vi "Start Sync.vi"(8 "error in (no error)":errorcluster, 11 "gRPC Server in":refnum<class "GreeterService.lvclass">) -> (0 "error out":errorcluster, 3 "gRPC Server out":refnum<class "GreeterService.lvclass">)   [LabVIEW 2019, in "Generated_server.lvlib" / "GreeterService.lvclass"]
uses:
  GreeterService.lvclass
  GreeterService.lvclass/GreeterService.ctl
  RPC Messages/Greeter_res.ctl
  RPC Messages/Greeter_res_res_oneof/Greeter_res_res_oneof.lvclass
  RPC Messages/Greeter_req_req_oneof/Greeter_req_req_oneof.lvclass/Greeter_req_req_oneof.ctl
  RPC Messages/Greeter_res_res_oneof/Greeter_res_res_oneof.lvclass/Greeter_res_res_oneof.ctl
  Generated_server.lvlib
  RPC Messages/Greeter_req_req_oneof/Greeter_req_req_oneof.lvclass
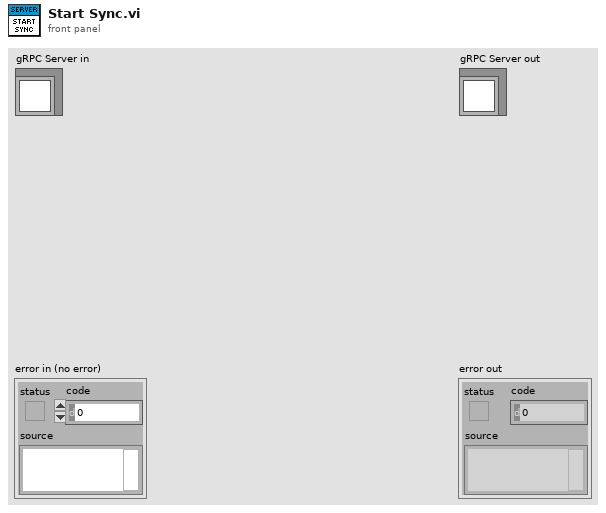
[diagram p1: front panel]
types:
  T1 = typedef "Generated_server.lvlib/Greeter_res.ctl" = cluster{"res_latitude":i32, "Greeter_res_res_oneof":refnum<class "Greeter_res_res_oneof.lvclass">}
  T2 = typedef "Generated_server.lvlib/GreeterService.lvclass/Server Internal UEs.ctl" = cluster{"GreeterService GetFeature Internal UE":refnum<user-event>}
  T3 = typedef "Generated_server.lvlib/GreeterService.lvclass/Server gRPC UEs.ctl" = cluster{"GreeterService GetFeature gRPC UE":refnum<user-event>}
  T4 = typedef "grpc-lvsupport-release.lvlib/grpcId.ctl" = u64
  T5 = typedef "Generated_server.lvlib/Greeter_req.ctl" = cluster{"req_latitude":i32, "Greeter_req_req_oneof":refnum<class "Greeter_req_req_oneof.lvclass">}
  T6 = typedef "grpc-lvsupport.lvlib/grpcId.ctl" = u64
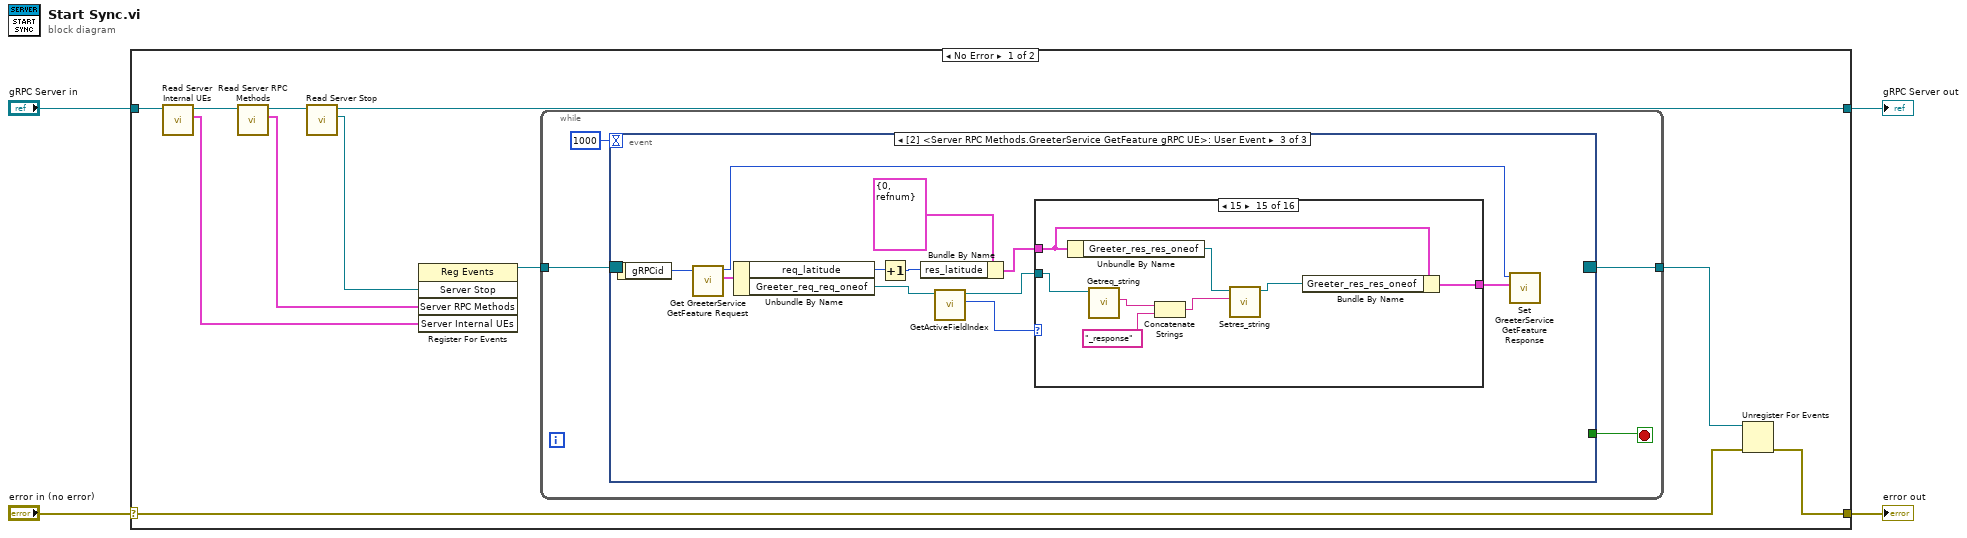
[diagram p0: block diagram]
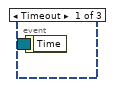
[diagram p2: hidden frame]
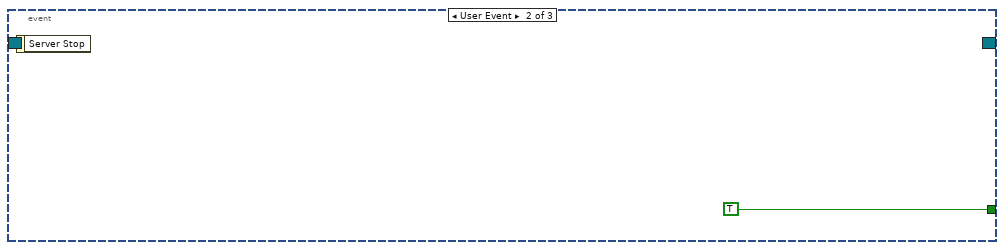
[diagram p3: hidden frame]
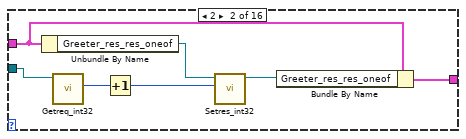
[diagram p5: hidden frame]
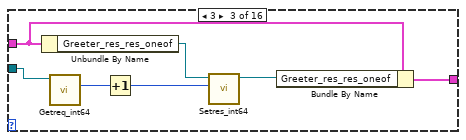
[diagram p6: hidden frame]
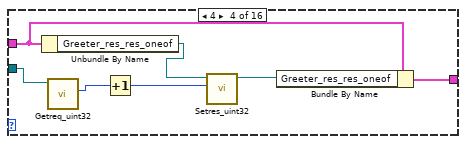
[diagram p7: hidden frame]
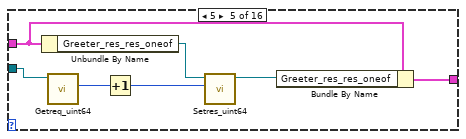
[diagram p8: hidden frame]
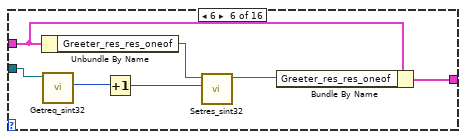
[diagram p9: hidden frame]
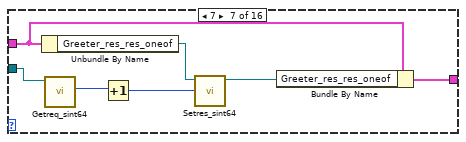
[diagram p10: hidden frame]
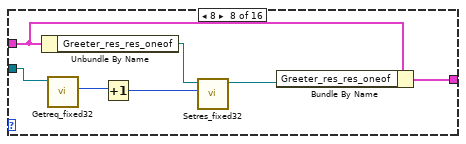
[diagram p11: hidden frame]
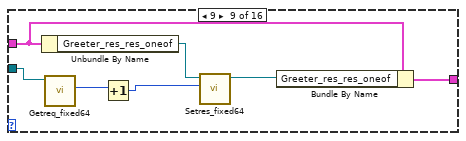
[diagram p12: hidden frame]
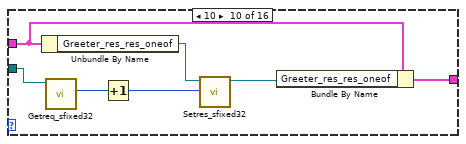
[diagram p13: hidden frame]
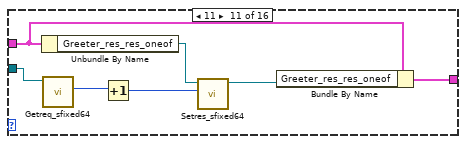
[diagram p14: hidden frame]
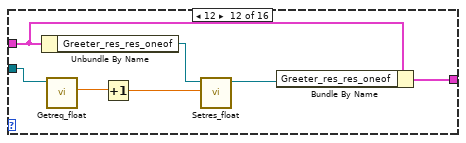
[diagram p15: hidden frame]
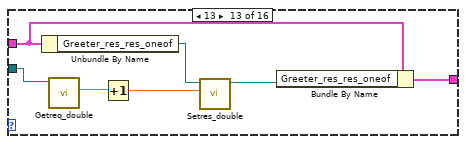
[diagram p16: hidden frame]
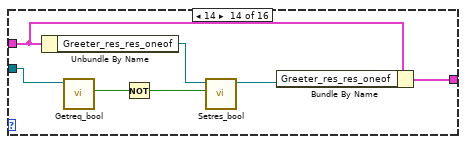
[diagram p17: hidden frame]
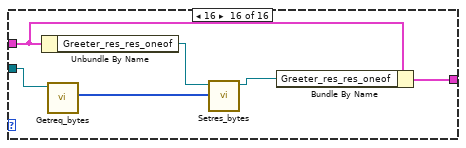
[diagram p18: hidden frame]
diagram:
  n1 = case shown="No Error" "error in (no error)" {
    selector: "error in (no error)" -> [w9 w139]
    tunnel: [w8 w139] -> w3
    tunnel: [w6 w138] -> w1
    tunnel: "gRPC Server in" -> [w15 w138]
    frame No Error {
      n2 = call "Read Server Internal UEs.vi"("SignalGeneratorService in"=w15) -> ("Server Internal UEs"=w13:T2, "SignalGeneratorService out"=w14:refnum<class "GreeterService.lvclass">)  [unwired: 8 in, 1 out]
      n3 = call "Read Server RPC Methods.vi"("SignalGeneratorService in"=w14) -> ("Server RPC Methods"=w7:T3, "SignalGeneratorService out"=w12:refnum<class "GreeterService.lvclass">)  [unwired: 8 in, 1 out]
      n4 = call-dynamic "Read Server Stop.vi"("iService in"=w12) -> ("Server Stop"=w5:refnum<user-event>, "iService out"=w6:refnum<class "GreeterService.lvclass">)  [unwired: 8 in, 1 out]
      n5 = register-events(w5, w7, w13) -> (reference out=w11:refnum<event-registration>)  [unwired: 2 in, 1 out]
      n6 = while {
        tunnel: w11 -> [w19]
        tunnel: [w17] -> w10
        stop <- w18 stop-if-true
        n7 = event "RPC Methods Event Structure" shown="[2] <Server RPC Methods.GreeterService GetFeature gRPC UE>: User Event" {
          selector: w19 -> [_ _ _]
          dyn-events: [_ _ _] -> w17
          timeout: 1000 -> [_ _ _]
          tunnel: [_ TRUE _] -> w18
          event Timeout {
            n8 = event-data() -> ()  [unwired: 1 in, 1 out]
          }
          event User Event {
            n9 = event-data() -> ()  [unwired: 1 in, 1 out]
          }
          event User Event {
            n10 = event-data() -> ("gRPCid"=w31:T4)  [unwired: 1 in]
            n11 = call "Get GreeterService GetFeature Request.vi"("gRPCid in"=w31) -> ("Message Data"=w30:T5, "gRPCid out"=w21:T6)  [unwired: 8 in, 1 out]
            n12 = Unbundle By Name(w30) -> ("req_latitude"=w27:i32, "Greeter_req_req_oneof"=w26:refnum<class "Greeter_req_req_oneof.lvclass">)
            n13 = Increment(x=w27) -> (x+1=w28:i32)
            n14 = Bundle By Name(cluster=T1 {"res_latitude"=0, "Greeter_res_res_oneof"=refnum} ("Greeter_res"), "res_latitude"=w28) -> (w24:T1)
            n15 = call "GetActiveFieldIndex.vi"("OneOfTemplate in"=w26) -> ("Active Field Index"=w25:i32, "OneOfTemplate out"=w23:refnum<class "Greeter_req_req_oneof.lvclass">)  [unwired: 8 in, 1 out]
            n16 = case shown="15" w25 {
              tunnel: w24 -> [w32 w35 w46 w53 w60 w67 w74 w81 w88 w95 w102 w109 w116 w123 w131 w137]
              tunnel: w23 -> [_ w39 w44 w51 w58 w65 w72 w79 w86 w93 w98 w107 w114 w121 w129 w135]
              tunnel: [w32 w33 w45 w52 w59 w66 w73 w80 w87 w94 w101 w108 w115 w122 w130 w136] -> w22
              frame 0, Default {
              }
              frame 2 {
                n17 = Unbundle By Name(w35) -> ("Greeter_res_res_oneof"=w36:refnum<class "Greeter_res_res_oneof.lvclass">)
                n18 = call "Getreq_int32.vi"("OneOfTemplate in"=w39) -> ("Get_Val"=w38:i32)  [unwired: 8 in, 2 out]
                n19 = Increment(x=w38) -> (x+1=w37:i32)
                n20 = call "Setres_int32.vi"("Set_Val"=w37, "OneOfTemplate in"=w36) -> ("OneOfTemplate out"=w34:refnum<class "Greeter_res_res_oneof.lvclass">)  [unwired: 8 in, 1 out]
                n21 = Bundle By Name(cluster=w35, "Greeter_res_res_oneof"=w34) -> (w33:T1)
              }
              frame 3 {
                n22 = Unbundle By Name(w46) -> ("Greeter_res_res_oneof"=w42:refnum<class "Greeter_res_res_oneof.lvclass">)
                n23 = call "Getreq_int64.vi"("OneOfTemplate in"=w44) -> ("Get_Val"=w43:i64)  [unwired: 8 in, 2 out]
                n24 = Increment(x=w43) -> (x+1=w41:i64)
                n25 = call "Setres_int64.vi"("Set_Val"=w41, "OneOfTemplate in"=w42) -> ("OneOfTemplate out"=w40:refnum<class "Greeter_res_res_oneof.lvclass">)  [unwired: 8 in, 1 out]
                n26 = Bundle By Name(cluster=w46, "Greeter_res_res_oneof"=w40) -> (w45:T1)
              }
              frame 4 {
                n27 = Unbundle By Name(w53) -> ("Greeter_res_res_oneof"=w48:refnum<class "Greeter_res_res_oneof.lvclass">)
                n28 = call "Getreq_uint32.vi"("OneOfTemplate in"=w51) -> ("Get_Val"=w50:u32)  [unwired: 8 in, 2 out]
                n29 = Increment(x=w50) -> (x+1=w49:u32)
                n30 = call "Setres_uint32.vi"("Set_Val"=w49, "OneOfTemplate in"=w48) -> ("OneOfTemplate out"=w47:refnum<class "Greeter_res_res_oneof.lvclass">)  [unwired: 8 in, 1 out]
                n31 = Bundle By Name(cluster=w53, "Greeter_res_res_oneof"=w47) -> (w52:T1)
              }
              frame 5 {
                n32 = Unbundle By Name(w60) -> ("Greeter_res_res_oneof"=w55:refnum<class "Greeter_res_res_oneof.lvclass">)
                n33 = call "Getreq_uint64.vi"("OneOfTemplate in"=w58) -> ("Get_Val"=w57:u64)  [unwired: 8 in, 2 out]
                n34 = Increment(x=w57) -> (x+1=w56:u64)
                n35 = call "Setres_uint64.vi"("Set_Val"=w56, "OneOfTemplate in"=w55) -> ("OneOfTemplate out"=w54:refnum<class "Greeter_res_res_oneof.lvclass">)  [unwired: 8 in, 1 out]
                n36 = Bundle By Name(cluster=w60, "Greeter_res_res_oneof"=w54) -> (w59:T1)
              }
              frame 6 {
                n37 = Unbundle By Name(w67) -> ("Greeter_res_res_oneof"=w62:refnum<class "Greeter_res_res_oneof.lvclass">)
                n38 = call "Getreq_sint32.vi"("OneOfTemplate in"=w65) -> ("Get_Val"=w64:i32)  [unwired: 8 in, 2 out]
                n39 = Increment(x=w64) -> (x+1=w63:i32)
                n40 = call "Setres_sint32.vi"("Set_Val"=w63, "OneOfTemplate in"=w62) -> ("OneOfTemplate out"=w61:refnum<class "Greeter_res_res_oneof.lvclass">)  [unwired: 8 in, 1 out]
                n41 = Bundle By Name(cluster=w67, "Greeter_res_res_oneof"=w61) -> (w66:T1)
              }
              frame 7 {
                n42 = Unbundle By Name(w74) -> ("Greeter_res_res_oneof"=w69:refnum<class "Greeter_res_res_oneof.lvclass">)
                n43 = call "Getreq_sint64.vi"("OneOfTemplate in"=w72) -> ("Get_Val"=w71:i64)  [unwired: 8 in, 2 out]
                n44 = Increment(x=w71) -> (x+1=w70:i64)
                n45 = call "Setres_sint64.vi"("Set_Val"=w70, "OneOfTemplate in"=w69) -> ("OneOfTemplate out"=w68:refnum<class "Greeter_res_res_oneof.lvclass">)  [unwired: 8 in, 1 out]
                n46 = Bundle By Name(cluster=w74, "Greeter_res_res_oneof"=w68) -> (w73:T1)
              }
              frame 8 {
                n47 = Unbundle By Name(w81) -> ("Greeter_res_res_oneof"=w76:refnum<class "Greeter_res_res_oneof.lvclass">)
                n48 = call "Getreq_fixed32.vi"("OneOfTemplate in"=w79) -> ("Get_Val"=w78:u32)  [unwired: 8 in, 2 out]
                n49 = Increment(x=w78) -> (x+1=w77:u32)
                n50 = call "Setres_fixed32.vi"("Set_Val"=w77, "OneOfTemplate in"=w76) -> ("OneOfTemplate out"=w75:refnum<class "Greeter_res_res_oneof.lvclass">)  [unwired: 8 in, 1 out]
                n51 = Bundle By Name(cluster=w81, "Greeter_res_res_oneof"=w75) -> (w80:T1)
              }
              frame 9 {
                n52 = Unbundle By Name(w88) -> ("Greeter_res_res_oneof"=w83:refnum<class "Greeter_res_res_oneof.lvclass">)
                n53 = call "Getreq_fixed64.vi"("OneOfTemplate in"=w86) -> ("Get_Val"=w85:u64)  [unwired: 8 in, 2 out]
                n54 = Increment(x=w85) -> (x+1=w84:u64)
                n55 = call "Setres_fixed64.vi"("Set_Val"=w84, "OneOfTemplate in"=w83) -> ("OneOfTemplate out"=w82:refnum<class "Greeter_res_res_oneof.lvclass">)  [unwired: 8 in, 1 out]
                n56 = Bundle By Name(cluster=w88, "Greeter_res_res_oneof"=w82) -> (w87:T1)
              }
              frame 10 {
                n57 = Unbundle By Name(w95) -> ("Greeter_res_res_oneof"=w90:refnum<class "Greeter_res_res_oneof.lvclass">)
                n58 = call "Getreq_sfixed32.vi"("OneOfTemplate in"=w93) -> ("Get_Val"=w92:i32)  [unwired: 8 in, 2 out]
                n59 = Increment(x=w92) -> (x+1=w91:i32)
                n60 = call "Setres_sfixed32.vi"("Set_Val"=w91, "OneOfTemplate in"=w90) -> ("OneOfTemplate out"=w89:refnum<class "Greeter_res_res_oneof.lvclass">)  [unwired: 8 in, 1 out]
                n61 = Bundle By Name(cluster=w95, "Greeter_res_res_oneof"=w89) -> (w94:T1)
              }
              frame 11 {
                n62 = Unbundle By Name(w102) -> ("Greeter_res_res_oneof"=w97:refnum<class "Greeter_res_res_oneof.lvclass">)
                n63 = call "Getreq_sfixed64.vi"("OneOfTemplate in"=w98) -> ("Get_Val"=w100:i64)  [unwired: 8 in, 2 out]
                n64 = Increment(x=w100) -> (x+1=w99:i64)
                n65 = call "Setres_sfixed64.vi"("Set_Val"=w99, "OneOfTemplate in"=w97) -> ("OneOfTemplate out"=w96:refnum<class "Greeter_res_res_oneof.lvclass">)  [unwired: 8 in, 1 out]
                n66 = Bundle By Name(cluster=w102, "Greeter_res_res_oneof"=w96) -> (w101:T1)
              }
              frame 12 {
                n67 = Unbundle By Name(w109) -> ("Greeter_res_res_oneof"=w104:refnum<class "Greeter_res_res_oneof.lvclass">)
                n68 = call "Getreq_float.vi"("OneOfTemplate in"=w107) -> ("Get_Val"=w106:sgl)  [unwired: 8 in, 2 out]
                n69 = Increment(x=w106) -> (x+1=w105:sgl)
                n70 = call "Setres_float.vi"("Set_Val"=w105, "OneOfTemplate in"=w104) -> ("OneOfTemplate out"=w103:refnum<class "Greeter_res_res_oneof.lvclass">)  [unwired: 8 in, 1 out]
                n71 = Bundle By Name(cluster=w109, "Greeter_res_res_oneof"=w103) -> (w108:T1)
              }
              frame 13 {
                n72 = Unbundle By Name(w116) -> ("Greeter_res_res_oneof"=w111:refnum<class "Greeter_res_res_oneof.lvclass">)
                n73 = call "Getreq_double.vi"("OneOfTemplate in"=w114) -> ("Get_Val"=w113:dbl)  [unwired: 8 in, 2 out]
                n74 = Increment(x=w113) -> (x+1=w112:dbl)
                n75 = call "Setres_double.vi"("Set_Val"=w112, "OneOfTemplate in"=w111) -> ("OneOfTemplate out"=w110:refnum<class "Greeter_res_res_oneof.lvclass">)  [unwired: 8 in, 1 out]
                n76 = Bundle By Name(cluster=w116, "Greeter_res_res_oneof"=w110) -> (w115:T1)
              }
              frame 14 {
                n77 = Unbundle By Name(w123) -> ("Greeter_res_res_oneof"=w118:refnum<class "Greeter_res_res_oneof.lvclass">)
                n78 = call "Getreq_bool.vi"("OneOfTemplate in"=w121) -> ("Get_Val"=w120:bool)  [unwired: 8 in, 2 out]
                n79 = Not(x=w120) -> (.not. x?=w119:bool)
                n80 = call "Setres_bool.vi"("Set_Val"=w119, "OneOfTemplate in"=w118) -> ("OneOfTemplate out"=w117:refnum<class "Greeter_res_res_oneof.lvclass">)  [unwired: 8 in, 1 out]
                n81 = Bundle By Name(cluster=w123, "Greeter_res_res_oneof"=w117) -> (w122:T1)
              }
              frame 15 {
                n82 = Unbundle By Name(w131) -> ("Greeter_res_res_oneof"=w125:refnum<class "Greeter_res_res_oneof.lvclass">)
                n83 = call "Getreq_string.vi"("OneOfTemplate in"=w129) -> ("Get_Val"=w127:string)  [unwired: 8 in, 2 out]
                n84 = Concatenate Strings(w127, "_response" ("string")) -> (w126:string)
                n85 = call "Setres_string.vi"("Set_Val"=w126, "OneOfTemplate in"=w125) -> ("OneOfTemplate out"=w124:refnum<class "Greeter_res_res_oneof.lvclass">)  [unwired: 8 in, 1 out]
                n86 = Bundle By Name(cluster=w131, "Greeter_res_res_oneof"=w124) -> (w130:T1)
              }
              frame 16 {
                n87 = Unbundle By Name(w137) -> ("Greeter_res_res_oneof"=w133:refnum<class "Greeter_res_res_oneof.lvclass">)
                n88 = call "Getreq_bytes.vi"("OneOfTemplate in"=w135) -> ("Get_Val"=w134:u8[])  [unwired: 8 in, 2 out]
                n89 = call "Setres_bytes.vi"("Set_Val"=w134, "OneOfTemplate in"=w133) -> ("OneOfTemplate out"=w132:refnum<class "Greeter_res_res_oneof.lvclass">)  [unwired: 8 in, 1 out]
                n90 = Bundle By Name(cluster=w137, "Greeter_res_res_oneof"=w132) -> (w136:T1)
              }
            }
            n91 = call "Set GreeterService GetFeature Response.vi"("Message Data"=w22, "gRPCid in"=w21) -> ()  [unwired: 9 in, 1 out]
          }
        }
      }
      n92 = Unregister For Events(event registration refnum=w10, error in=w9) -> (error out=w8:errorcluster)
    }
    frame Error {
    }
  }
  "error out" <- w3
  "gRPC Server out" <- w1
